vi "Build Pulse Command.vi"(8 "error in":errorcluster, 9 "Pulse Enable":bool, 10 "Channel":i32, 11 "3300 in":refnum<class "3300.lvclass">) -> (0 "error out":errorcluster, 2 "Pulse Instruction":string, 3 "3300 out":refnum<class "3300.lvclass">)   [LabVIEW 2019, in "3300.lvlib" / "3300.lvclass"]
uses:
  Library/3300.lvclass
  C:/Users/Public/Documents/Development/builds/Instruments/Electronic Load.lvlibp/Library/Electronic Load.lvclass
  builds/Instruments/Electronic Load.lvlibp/Accessors/Trigger/Read Pulse Mode.vi
  builds/Instruments/Electronic Load.lvlibp/Accessors/Trigger/Read Pulse Initial.vi
  builds/Instruments/Electronic Load.lvlibp/Accessors/Trigger/Read Transient.vi
  builds/Instruments/Electronic Load.lvlibp/Accessors/Trigger/Read Pulse Width.vi
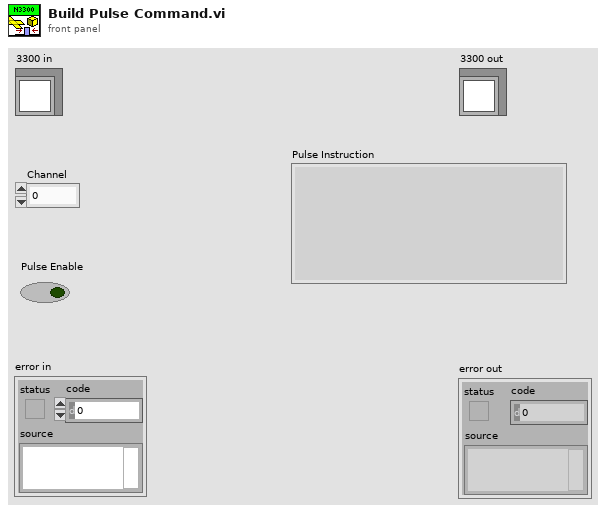
[diagram p1: front panel]
types:
  T1 = typedef "Electronic Load.lvlibp/Electronic Load.lvclass/E-Load Mode.ctl" = enum16{"Current", "Resistance", "Voltage"}
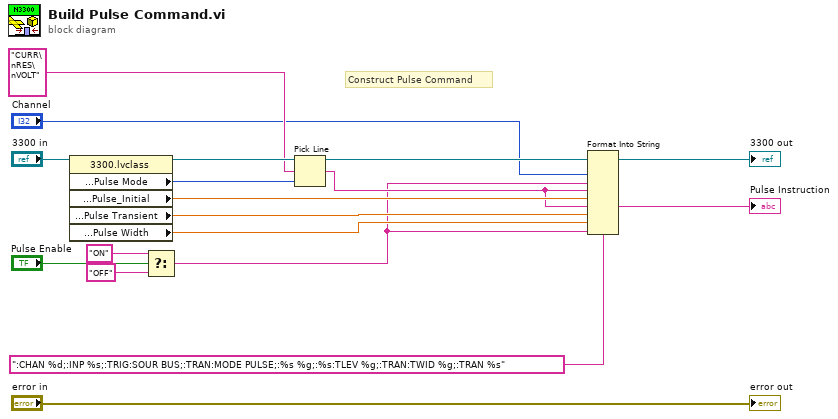
[diagram p0: block diagram]
diagram:
  # "Construct Pulse Command"
  n1 = property class="3300.lvclass"(reference="3300 in") -> (reference out=→"3300 out":refnum<class "3300.lvclass">, "Accessors:Settings:Pulse:Pulse Mode"=w13:T1, "Accessors:Settings:Pulse:Pulse_Initial"=w5:dbl, "Accessors:Settings:Pulse:Pulse Transient"=w4:dbl, "Accessors:Settings:Pulse:Pulse Width"=w3:dbl)  [unwired: 1 in, 1 out]
  n2 = Select(t="ON" ("Trig Enabled"), s="Pulse Enable", f="OFF" ("Trig Enabled")) -> (s? t:f=w1:string)
  n3 = Pick Line(multi-line string="CURR\nRES\nVOLT", line index=w13) -> (output string=w2:string)  [unwired: 1 in]
  n4 = Format Into String(format string=":CHAN %d;:INP %s;:TRIG:SOUR BUS;:TRAN:MODE PULSE;:%s %g;:%s:TLEV %g;:TRAN:TWID %g;:TRAN %s", "Channel", w1, w2, w5, w2, w4, w3, w1) -> (resulting string=→"Pulse Instruction":string)  [unwired: 2 in, 1 out]
  "error out" <- "error in"
